vi "DATA S CURVE.vi"(0 "Distância Guias (um)":dbl=50.0, 1 "Distância Ac (um)":dbl=50.0, 2 "Raio":dbl=7.0, 3 "Xc":dbl=2.0, 4 "Blank Button":bool) -> (5 "1st curve":cluster{"Yc":dbl, "Xc":dbl, "Angle":dbl}, 6 "2nd curve":cluster{"Yc":dbl, "Xc":dbl, "Angle":dbl})   [LabVIEW 2014]
panel:
  # "ACESSO: CURVAS TIPO 1\nAPAGADO: CURVAS TIPO 2"
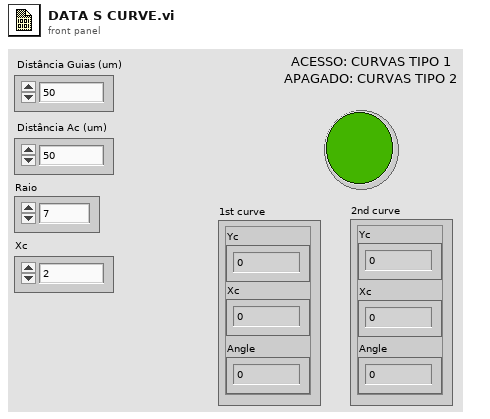
[diagram p1: front panel]
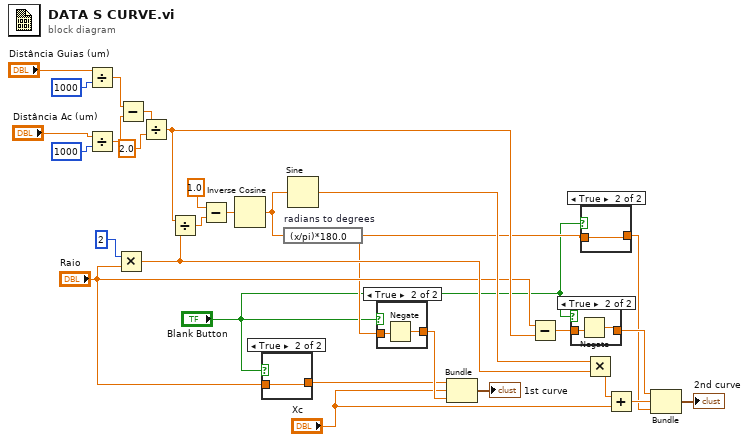
[diagram p0: block diagram]
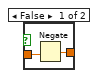
[diagram p2: hidden frame]
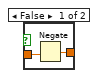
[diagram p4: hidden frame]
diagram:
  n1 = Divide(x="Distância Guias (um)", y=1000) -> (x/y=w16:dbl)
  n2 = Divide(x="Distância Ac (um)", y=1000) -> (x/y=w15:dbl)
  n3 = Multiply(x=2 ("y"), y="Raio") -> (x*y=w27:dbl)
  n4 = Subtract(x=w16, y=w15) -> (x-y=w13:dbl)
  n5 = Divide(x=w13, y=2.0) -> (x/y=w11:dbl)
  n6 = Divide(x=w11, y=w27) -> (x/y=w21:dbl)
  n7 = Subtract(x=1.0, y=w21) -> (x-y=w23:dbl)
  n8 = Inverse Cosine(1:w23) -> (0:w24:dbl)
  n9 = case shown="True" "Blank Button" {
    tunnel: "Raio" -> [w31 w32]
    tunnel: [w30 w32] -> w10
    frame False {
      n10 = Negate(x=w31) -> (-x=w30:dbl)
    }
    frame True {
    }
  }
  n11 = expression code="(x/pi)*180.0" "radians to degrees"(w24) -> (w6:dbl)
  n12 = Sine(x=w24) -> (sin(x)=w28:dbl)
  n13 = case shown="True" "Blank Button" {
    tunnel: w6 -> [w33 w35]
    tunnel: [w33 w34] -> w14
    frame False {
    }
    frame True {
      n14 = Negate(x=w35) -> (-x=w34:dbl)
    }
  }
  n15 = Bundle("Raio"=w10, "Xc"="Xc", w14) -> (→"1st curve":cluster{"Raio":dbl, "Xc":dbl, dbl})  [unwired: 1 in]
  n16 = Subtract(x="Raio", y=w11) -> (x-y=w8:dbl)
  n17 = case shown="True" "Blank Button" {
    tunnel: w8 -> [w36 w38]
    tunnel: [w36 w37] -> w7
    frame False {
    }
    frame True {
      n18 = Negate(x=w38) -> (-x=w37:dbl)
    }
  }
  n19 = case shown="True" "Blank Button" {
    tunnel: w6 -> [w40 w41]
    tunnel: [w39 w41] -> w5
    frame False {
      n20 = Negate(x=w40) -> (-x=w39:dbl)
    }
    frame True {
    }
  }
  n21 = Multiply(x=w28, y=w27) -> (x*y=w25:dbl)
  n22 = Add(x=w25, y="Xc") -> (x+y=w26:dbl)
  n23 = Bundle(w7, w26, w5) -> (→"2nd curve":cluster{dbl, dbl, dbl})  [unwired: 1 in]
